vi "WriteToXML.vi"(8 "error in (no error)":errorcluster, 10 "Class Label":string="AzElParameters", 11 "AzElParameters in":refnum<class "AzElParameters.lvclass">) -> (0 "error out":errorcluster, 2 "XML out":string="<>\n  <azimuth>\n    <degreesArc>0</degreesArc>\n    <minutesArc>0</minutesArc>\n    <secondsArc>0</secondsArc>\n  </azimuth>\n  <elevation>\n    <degreesAlt>90</degreesAlt>\n    <minutesArc>0</minutesArc>\n    <secondsArc>0</secondsArc>\n  </elevation>\n</>", 3 "AzElParameters out":refnum<class "AzElParameters.lvclass">)   [LabVIEW 2014, in "TCSDataDefinitions.lvlib" / "TCSCommand.lvlib" / "TargetConfiguration.lvlib" / "Target.lvlib" / "FixedTarget.lvlib" / "AzElParameters.lvclass"]
uses:
  AzElParameters.lvclass
  AzElParameters.lvclass/AzElParameters.ctl
  Azimuth/Azimuth.lvclass
  Elevation/Elevation.lvclass
  <userlib>/Common/XML/XMLGenerator/XMLGenerator.lvclass
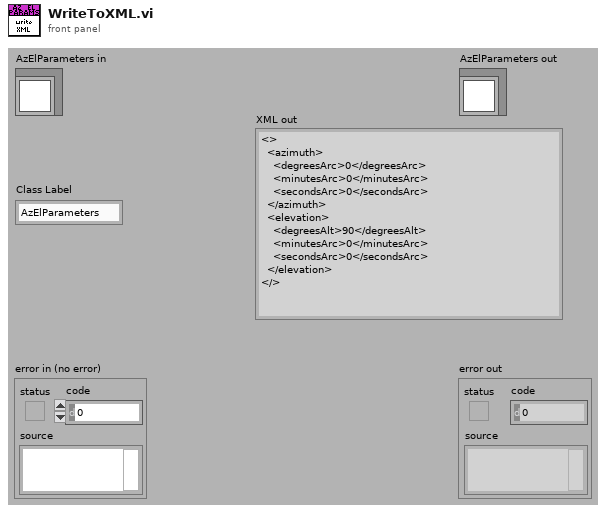
[diagram p1: front panel]
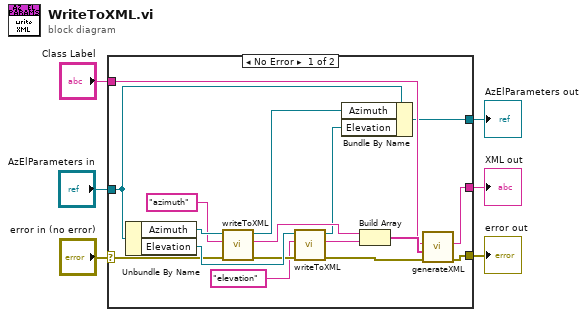
[diagram p0: block diagram]
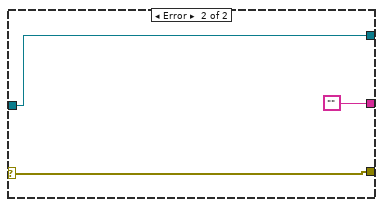
[diagram p2: hidden frame]
diagram:
  n1 = case shown="No Error" "error in (no error)" {
    selector: "error in (no error)" -> [w20 w26]
    tunnel: [w11 w26] -> w5
    tunnel: [w10 w25] -> w3
    tunnel: "AzElParameters in" -> [w9 w25]
    tunnel: "Class Label" -> [w14 _]
    tunnel: [w13 ""] -> w1
    frame No Error {
      n2 = Unbundle By Name(w9) -> ("Azimuth"=w22:refnum<class "Azimuth.lvclass">, "Elevation"=w23:refnum<class "Elevation.lvclass">)
      n3 = call-dynamic "writeToXML.vi"("error in (no error)"=w20, "Class Label"="azimuth", "Azimuth in"=w22) -> ("error out"=w21:errorcluster, "XML out"=w17:string, "Azimuth out"=w8:refnum<class "Azimuth.lvclass">)  [unwired: 6 in]
      n4 = call-dynamic "writeToXML.vi"("error in (no error)"=w21, "Class Label"="elevation", "Elevation in"=w23) -> ("error out"=w12:errorcluster, "XML out"=w16:string, "Elevation out"=w7:refnum<class "Elevation.lvclass">)  [unwired: 6 in]
      n5 = Bundle By Name(cluster=w9, "Azimuth"=w8, "Elevation"=w7) -> (w10:refnum<class "AzElParameters.lvclass">)
      n6 = Build Array(w17, w16) -> (w15:string[])
      n7 = call <userlib>:"generateXML.vi"("error in"=w12, "childrenXML"=w15, "elementName"=w14) -> ("error out"=w11:errorcluster, "XML out"=w13:string)  [unwired: 6 in, 1 out]
    }
    frame Error {
    }
  }
  "error out" <- w5
  "AzElParameters out" <- w3
  "XML out" <- w1
